vi "Save Cp snapshot.vi"(0 "Pdyn ref (Pa)":sgl, 1 "rho ref (kg/m^3)":sgl, 2 "radius (m)":sgl=0.02858, 3 "span (m)":sgl=0.43, 4 "Fx (N)":sgl, 5 "Fy (N)":sgl, 6 "Cp distribution (time averaged)":cluster{"x/c flap (sorted)":sgl[], sgl[]}[](graph), 8 "d.p":i16=4, 10 "File Path":path=path "C:/Datalogs/Cp snapshot 001.txt") -> (19 "error out":errorcluster)   [LabVIEW 2015]
uses:
  <vilib>/Utility/file.llb/Write Delimited Spreadsheet (string).vi
panel:
  in  "y/c cylinder":sgl[](array[numeric])=[0.25881904, 0.5, 0.70710677, 0.8660254, 0.9659258, 0.9659258, 0.8660254, 0.70710677, 0.5, 0.25881904, -0.25881904, -0.5, -0.70710677, -0.8660254, -0.9659258, -0.9659258, -0.8660254, -0.70710677, -0.5, -0.25881904]
  # "Paste in values from Geometry Prep vi"
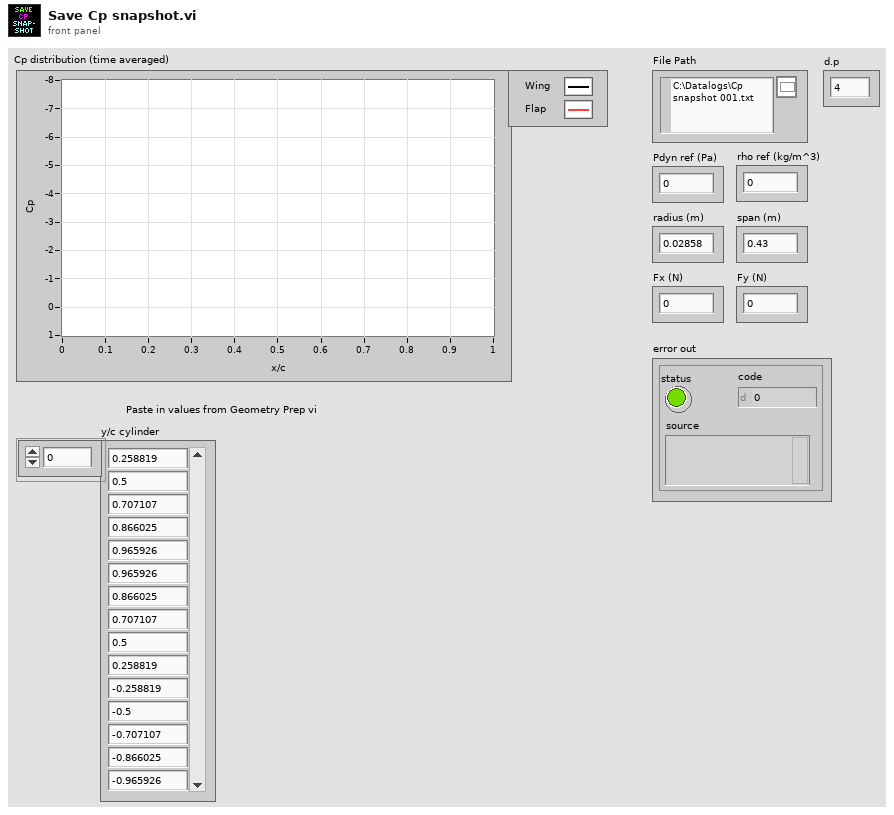
[diagram p1: front panel]
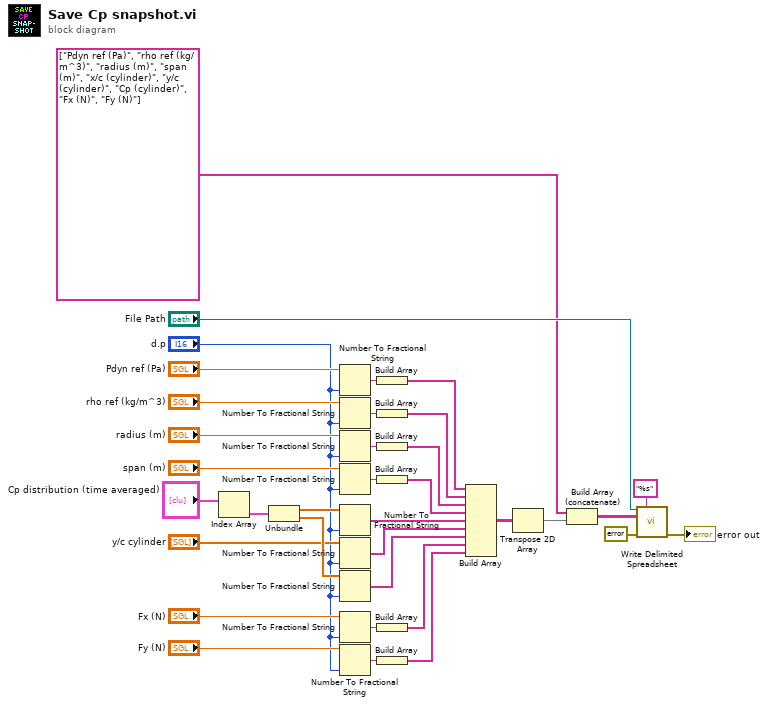
[diagram p0: block diagram]
diagram:
  n1 = Index Array(array="Cp distribution (time averaged)") -> (element=w34:cluster{"x/c flap (sorted)":sgl[], sgl[]})  [unwired: 1 in]
  n2 = Unbundle(w34) -> ("x/c flap (sorted)"=w33:sgl[], w32:sgl[])
  n3 = Number To Fractional String(number="Pdyn ref (Pa)", precision (6)="d.p") -> (F-format string=w21:string)  [unwired: 2 in]
  n4 = Number To Fractional String(number="rho ref (kg/m^3)", precision (6)="d.p") -> (F-format string=w13:string)  [unwired: 2 in]
  n5 = Number To Fractional String(number="radius (m)", precision (6)="d.p") -> (F-format string=w8:string)  [unwired: 2 in]
  n6 = Number To Fractional String(number="span (m)", precision (6)="d.p") -> (F-format string=w7:string)  [unwired: 2 in]
  n7 = Number To Fractional String(number=w33, precision (6)="d.p") -> (F-format string=w31:string[])  [unwired: 2 in]
  n8 = Number To Fractional String(number="y/c cylinder", precision (6)="d.p") -> (F-format string=w2:string[])  [unwired: 2 in]
  n9 = Number To Fractional String(number=w32, precision (6)="d.p") -> (F-format string=w3:string[])  [unwired: 2 in]
  n10 = Number To Fractional String(number="Fx (N)", precision (6)="d.p") -> (F-format string=w18:string)  [unwired: 2 in]
  n11 = Number To Fractional String(number="Fy (N)", precision (6)="d.p") -> (F-format string=w17:string)  [unwired: 2 in]
  n12 = Build Array(w21) -> (w12:string[])
  n13 = Build Array(w13) -> (w11:string[])
  n14 = Build Array(w8) -> (w6:string[])
  n15 = Build Array(w7) -> (w5:string[])
  n16 = Build Array(w18) -> (w16:string[])
  n17 = Build Array(w17) -> (w15:string[])
  n18 = Build Array(w12, w11, w6, w5, w31, w2, w3, w16, w15) -> (w30:string[][])
  n19 = Transpose 2D Array(2D array=w30) -> (transposed array=w29:string[][])
  n20 = Build Array (concatenate)(string[] ["Pdyn ref (Pa)", "rho ref (kg/m^3)", "radius (m)", "span (m)", "x/c (cylinder)", "y/c (cylinder)", "Cp (cylinder)", "Fx (N)", "Fy (N)"], w29) -> (w28:string[][])
  n21 = call-poly <vilib>:"Write Delimited Spreadsheet.vi"("file path (dialog if empty)"="File Path", "format (%s)"="%s", "2D data"=w28, "error in (no error)"=errorcluster {"status"=FALSE, "code"=0, "source"=""}) -> ("error out"=→"error out":errorcluster)  [unwired: 10 in, 1 out]
